vi "Event Destroy.vi"(8 "error in (no error)":errorcluster, 11 "Event DVR in":refnum<data-value>) -> (0 "error out":errorcluster)   [LabVIEW 2010, in "MDSplus.lvlib"]
uses:
  <vilib>/MDSplus/Library/MDSplus.lvlib
  <vilib>/MDSplus/Classes/Event_Class/Event.lvclass
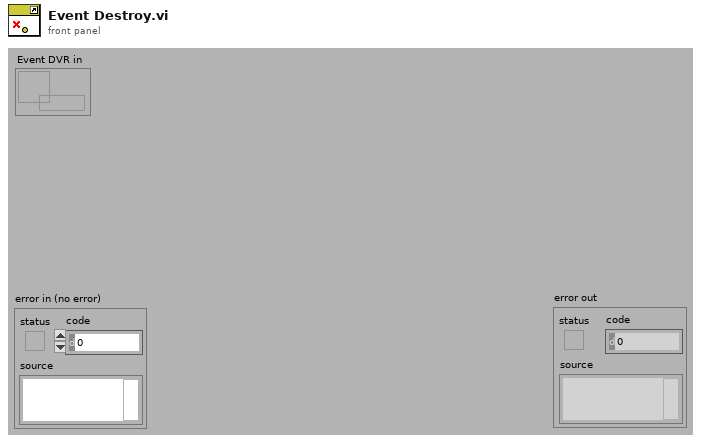
[diagram p1: front panel]
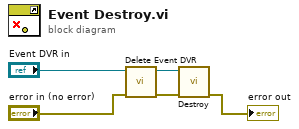
[diagram p0: block diagram]
diagram:
  n1 = call <vilib>:"Delete Event DVR.vi"("error in (no error)"="error in (no error)", "Event DVR in"="Event DVR in") -> ("error out"=w2:errorcluster, "Event out"=w3:refnum<class "Event.lvclass">)  [unwired: 8 in]
  n2 = call-dynamic "Destroy.vi"("error in (no error)"=w2, "Event in"=w3) -> ("error out"=→"error out":errorcluster)  [unwired: 9 in]
